vi "Smart IO Get Analog Voltage.vi"(8 "error in (no error)":errorcluster, 11 "deviceIndex":i32=-1) -> (0 "error out":errorcluster, 1 "Raw Value":u32, 2 "Voltage":dbl)   [LabVIEW 2026, in "MrcLib.lvlib"]
doc: "Returns the voltage value directly from the A/D converter on the channel. The converter scales the raw value to the voltage value using the least significant bit weight constant and the offset constant of the hardware."
uses:
  MrcLib.lvlib
  Types/MRC Smart IO Mode.ctl
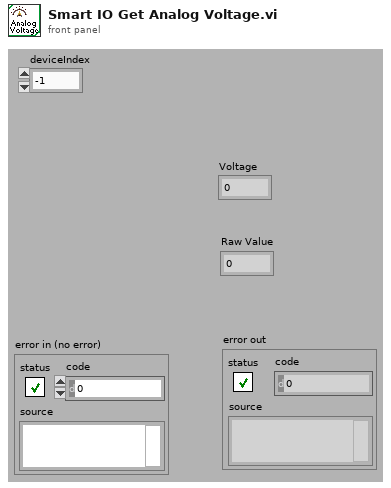
[diagram p1: front panel]
types:
  T1 = typedef "MRC Smart IO Mode.ctl" = i32
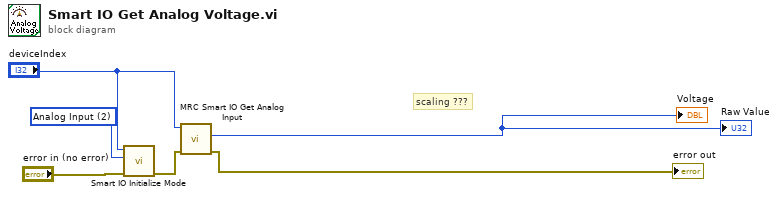
[diagram p0: block diagram]
diagram:
  w1 = T1 2 items=["Digital Input"=0, "Digital Output"=1, "Analog Input"=2, "PWM Input"=3, "PWM Output"=4, "Counter Rising"=5, "Counter Falling"=6, "Addressable LEDs"=13] ("mode")
  # "scaling ???"
  n1 = call "Smart IO Initialize Mode.vi"("error in (no error)"="error in (no error)", "mode"=w1, "deviceIndex"="deviceIndex") -> ("error out"=w3:errorcluster)  [unwired: 8 in]
  n2 = call "MRC Smart IO Get Analog Input.vi"("error in (no error)"=w3, "deviceIndex"="deviceIndex") -> ("error out"=→"error out":errorcluster, "value out"=→"Voltage" →"Raw Value":i32)  [unwired: 8 in]
